vi "WaveStablizer.vi"() -> ()   [LabVIEW 2014]
panel:
  in  "Data":dbl[][](array[numeric])
  in  "Buffer":i64
  out "Waveform Chart":dbl(graph)
  in  "Location":dbl[][](array[numeric])
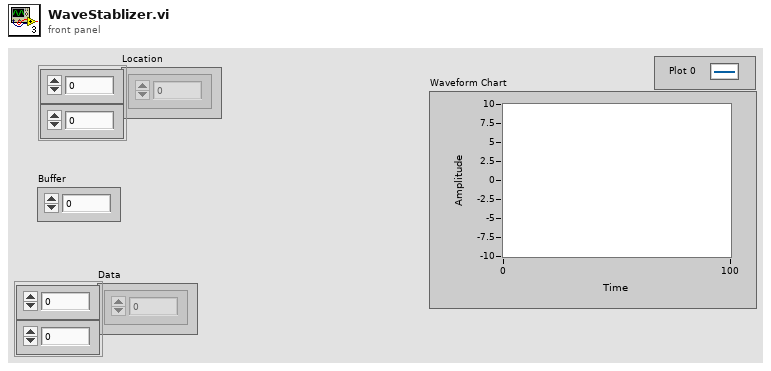
[diagram p1: front panel]
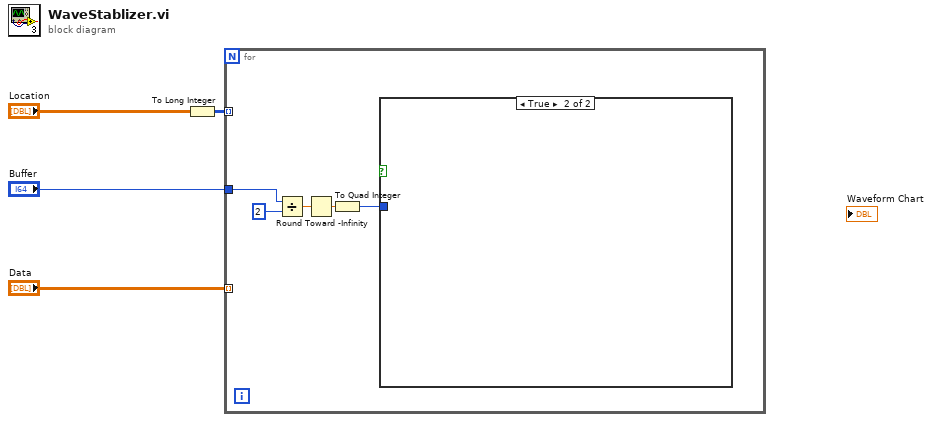
[diagram p0: block diagram]
diagram:
  n1 = To Long Integer(number="Location") -> (32bit integer=w3:i32[][])
  n2 = for {
    tunnel: w3 -> [_] mode=indexing
    tunnel: "Data" -> [_] mode=indexing
    tunnel: "Buffer" -> [w6]
    n3 = Divide(x=w6, y=i64 2) -> (x/y=w8:dbl)
    n4 = Round Toward -Infinity(1:w8) -> (0:w7:dbl)
    n5 = To Quad Integer(1:w7) -> (0:w5:i64)
    n6 = case shown="True" {
      selector: _ -> [_ _]
      tunnel: w5 -> [_ _]
      frame False {
      }
      frame True {
      }
    }
  }
